vi "ble_reset_dongle_and_cnx.vi"(8 "error in (no error)":errorcluster, 9 "Reset?":bool, 10 "wait time (100)":u32=1000, 11 "COM Bluegiga in":refnum<visa-resource-name>) -> (0 "error out":errorcluster, 3 "COM Bluegiga out":refnum<visa-resource-name>)   [LabVIEW 2015]
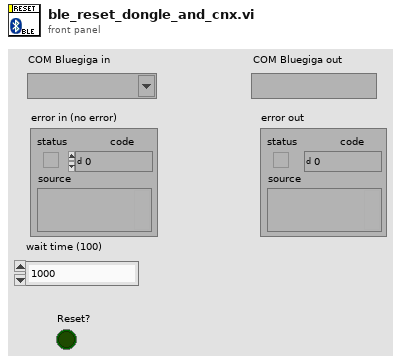
[diagram p1: front panel]
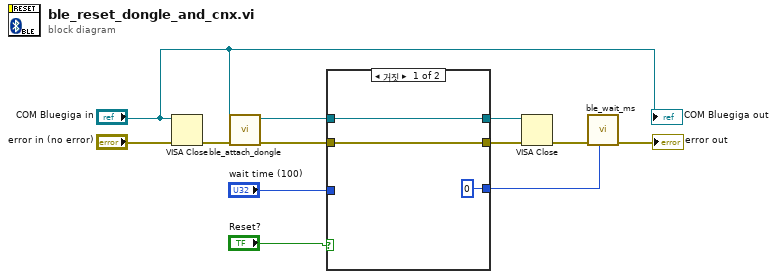
[diagram p0: block diagram]
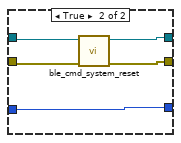
[diagram p2: hidden frame]
diagram:
  n1 = VISA Close(VISA resource name="COM Bluegiga in", error in (no error)="error in (no error)") -> (error out=w7:errorcluster)
  n2 = call "ble_attach_dongle.vi"("error in (no error)"=w7, "COM Bluegiga in"="COM Bluegiga in") -> ("error out"=w8:errorcluster, "COM Bluegiga out"=w9:refnum<visa-resource-name>)  [unwired: 8 in]
  n3 = case shown="거짓" "Reset?" {
    tunnel: [w15 w20] -> w11
    tunnel: [w14 w19] -> w10
    tunnel: w9 -> [w15 w18]
    tunnel: w8 -> [w14 w17]
    tunnel: [u32 0 ("wait time (100)") w16] -> w2
    tunnel: "wait time (100)" -> [_ w16]
    frame False {
    }
    frame True {
      n4 = call "ble_cmd_system_reset.vi"("error in (no error)"=w17, "COM Bluegiga in"=w18) -> ("error out"=w19:errorcluster, "COM Bluegiga out"=w20:refnum<visa-resource-name>)  [unwired: 8 in]
    }
  }
  n5 = VISA Close(VISA resource name=w11, error in (no error)=w10) -> (error out=w12:errorcluster)
  n6 = call "ble_wait_ms.vi"("milliseconds to wait (100)"=w2, "error in (no error)"=w12) -> ("error out"=→"error out":errorcluster)  [unwired: 9 in]
  "COM Bluegiga out" <- "COM Bluegiga in"
